vi "From Serial Form.vi"(6 "Serial Version":T1, 10 "Deserializer in":refnum<class "Deserializer.lvclass">, 11 "Single_Array in":refnum<class "Single_Array.lvclass">) -> (0 "error out":errorcluster, 2 "Deserializer out":refnum<class "Deserializer.lvclass">, 3 "Single_Array out":refnum<class "Single_Array.lvclass">)   [LabVIEW 2014, in "Base Data Class.lvlib" / "Single_Array.lvclass"]
uses:
  Single_Array.lvclass
  <vilib>/NI/AQ Character Lineator/Deserializer/Deserializer.lvclass
  <vilib>/NI/AQ Character Lineator/Serialization Common/Serial Version.ctl
  Single_Array.lvclass/Single_Array.ctl
  <vilib>/NI/AQ Character Lineator/Serializable/Remove Single Array.vi
  Data.lvclass
  <vilib>/NI/AQ Character Lineator/Serializable/Serializable.lvclass
  <vilib>/NI/AQ Character Lineator/Serialization Common/Serialization Common.lvlib
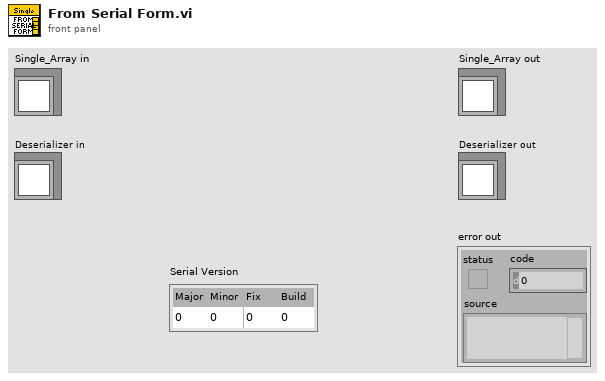
[diagram p1: front panel]
types:
  T1 = typedef "Serialization Common.lvlib/Serial Version.ctl" = cluster{"Major":u16, "Minor":u16, "Fix":u16, "Build":u16}
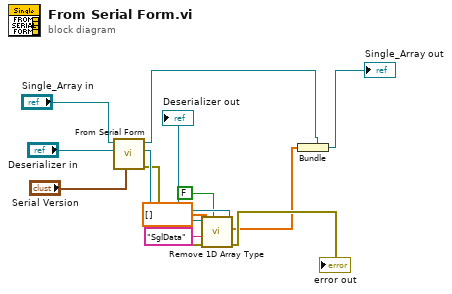
[diagram p0: block diagram]
diagram:
  n1 = call-parent "From Serial Form.vi"("Serial Version"="Serial Version", "Deserializer in"="Deserializer in", "Data in"="Single_Array in") -> ("error out"=w9:errorcluster, "Deserializer out"=w10:refnum<class "Deserializer.lvclass">, "Data out"=w5:refnum<class "Single_Array.lvclass">)  [unwired: 6 in]
  n2 = call-poly <vilib>:"Remove 1D Array Type.vi"("Return Default Value Regardless (F)"=FALSE, "error in (no error)"=w9, "Name"="SglData", "Default Value"=sgl[] [], "Deserializer in"=w10) -> ("error out"=→"error out":errorcluster, "Singles"=w3:sgl[], "Deserializer out"=→"Deserializer out":refnum<class "Deserializer.lvclass">)  [unwired: 3 in, 1 out]
  n3 = Bundle(cluster=w5, w3) -> (→"Single_Array out":refnum<class "Single_Array.lvclass">)
